vi "Measurement UI.vi"() -> ()   [LabVIEW 2021, in "Crosstalk_Audio ADC_UI.lvlib"]
uses:
  Crosstalk_Audio ADC_UI.lvlib
  Program Files/National Instruments/LabVIEW 2021/examples/Digital Audio Acquisition and Generation Toolkit/subVIs/PCM Interface Type.ctl
  <vilib>/PDM Acquisition Toolkit/shared/controls/Digital Edge.ctl
  shared/Audio ADC Shared.lvlib
  <vilib>/PDM Acquisition Toolkit/shared/PDM Shared.lvlib
panel:
  out "MeasTable":string[][](table)
  in  "MeasGraphs":T1(tab)=enum."Time Domain"
  out "FreqDomainGraph":cluster{"f0":dbl, "df":dbl, dbl[]}(graph) caption="AC"
  out "TimeDomainGraph":waveform(dbl)(graph) caption="AC"
  out "Time domain plot size":i32
  out "Spectrum plot size":i32
  out "dt":dbl
  out "t0":dbl
  out "df":dbl
  out "f0":dbl
  out "Time domain":dbl[](array[numeric])
  out "Spectrum":dbl[](array[numeric])
  out "Crosstalk":dbl
  out "Victim channel name":string
  out "Crosstalk waveform":dbl[](array[numeric])
  out "Frequency waveform":dbl[](array[numeric])
  in  "Victim channel resource name":string
  in  "Digital capture resource name":string
  in  "Configuration tab":enum32{"Protocol", "Measurement"}(tab)
  in  "Frame sync edge for Channel 0":enum16{"Rising", "Falling"}(ring)=enum."Falling"
  in  "Channel count per frame":u8=2
  in  "Channel length":u16=32
  in  "Bit depth":u8=24
  in  "Channel 0 offset":u16=1
  in  "Endianness":enum16{"MSB First", "LSB First"}(ring)
  in  "Data Justification":enum16{"Left Justified", "Right Justified"}(ring) caption="Data justification"
  in  "Frame length":u16=64
  in  "Frame sync pulse width":u16=32
  in  "Bit clock edge sync":enum8{"Rising", "Falling"}(ring)=enum."Falling"
  in  "I2S":bool
  in  "LJ":bool
  in  "RJ":bool
  in  "TDM":bool
  in  "Measurement Duration":dbl=0.1 format="%#_6ps"
  in  "Analog source resource name":string(combo) caption="Resource Name"
  in  "Protocol capture resource name":string(combo) caption="Resource Name"
  in  "Channel Name":string
  in  "Full scale range":dbl=2.825 caption="FULL SCALE RANGE" format="%.3pV"
  in  "Weighting Filter":string(combo)="Linear"
  in  "Data line":u16 caption="Data Line"
  in  "Sample rate":dbl=44100.0 caption="Sample Rate" format="%#.6pHz"
  in  "Measurement settings":string="Measurement Settings"
  in  "Victim amplitude":dbl=1.0 caption="Amplitude" format="%#_6pdB"
  in  "Frequency":dbl=1000.0 format="%#_6pHz"
  in  "Victim channel":dbl=1.0 caption="Vicitim Channel" format="%#_6p"
  in  "Interferer channel":dbl caption="Interferer Channel" format="%#_6p"
  in  "Analog source":string="Analog source"
  in  "Digital capture":string="Digital capture"
  # "Protocols"
  # "PCM data configuration"
  # "Frame sync clock control"
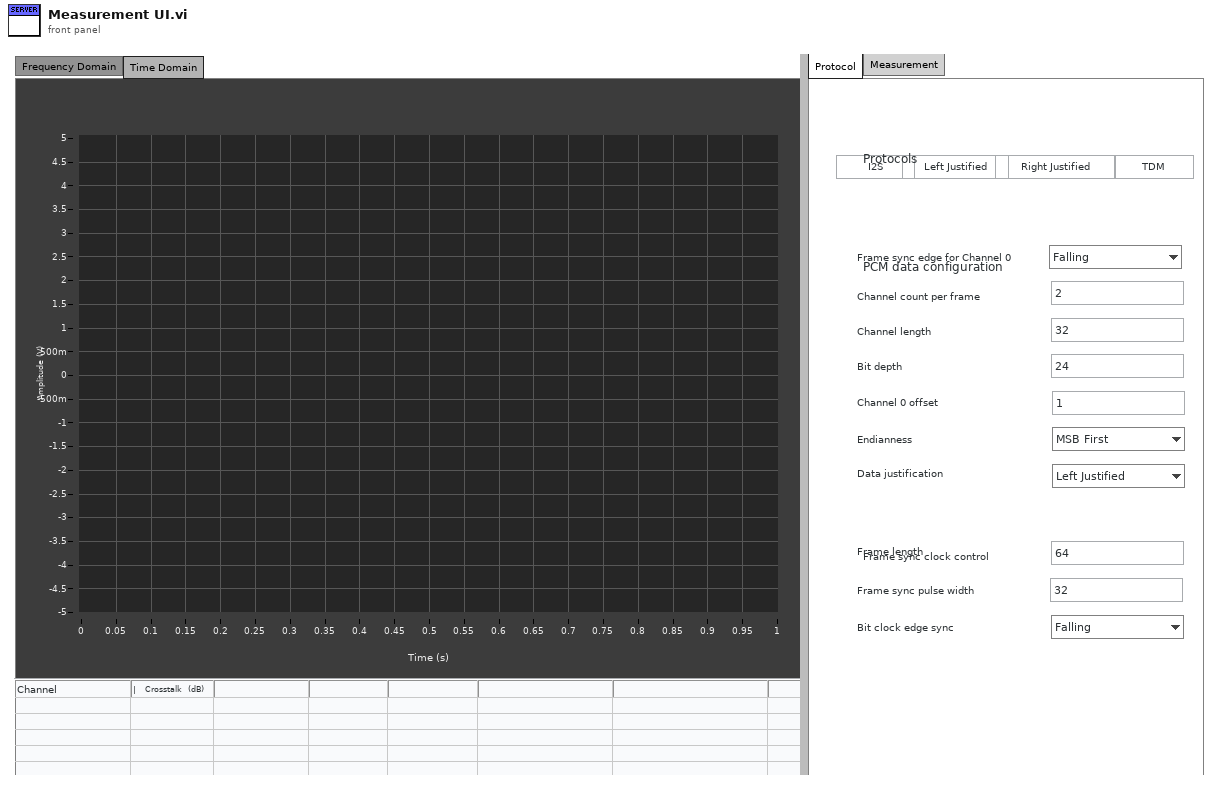
[diagram p1: front panel]
types:
  T1 = enum32{"Frequency Domain", "Time Domain", "Hidden Controls"}
  T2 = typedef "PDM Shared.lvlib/Digital Edge.ctl" = enum8{"Rising", "Falling"}
  T3 = typedef "PCM Interface Type.ctl" = enum16{"I2S", "Left Justified", "Right Justified", "TDM 4 Channel", "TDM 6 Channel", "TDM 8 Channel", "DSP mode", "DSP mode with 1 bit delay", "PCM Short Frame", "PCM Long Frame"}
  T4 = typedef "PDM Shared.lvlib/PCM Frame Sync Control.ctl" = cluster{"Frame Length":u16, "Frame Sync Pulse Width":u16, "Bit Clock Edge  Sync":T2}
  T5 = typedef "PDM Shared.lvlib/PCM Data Format Configuration.ctl" = cluster{"Frame Sync Edge for Channel 0":T2, "Channel Count Per Frame":u8, "Channel Length":u16, "Bit Depth":u8, "Channel 0 Offset":u16, "Endianness":T6, "Data Justification":T7}
  T6 = typedef "PDM Shared.lvlib/PCM Bit Endianness.ctl" = enum16{"MSB First", "LSB First"}
  T7 = typedef "PDM Shared.lvlib/PCM Data Justification.ctl" = enum16{"Left Justified", "Right Justified"}
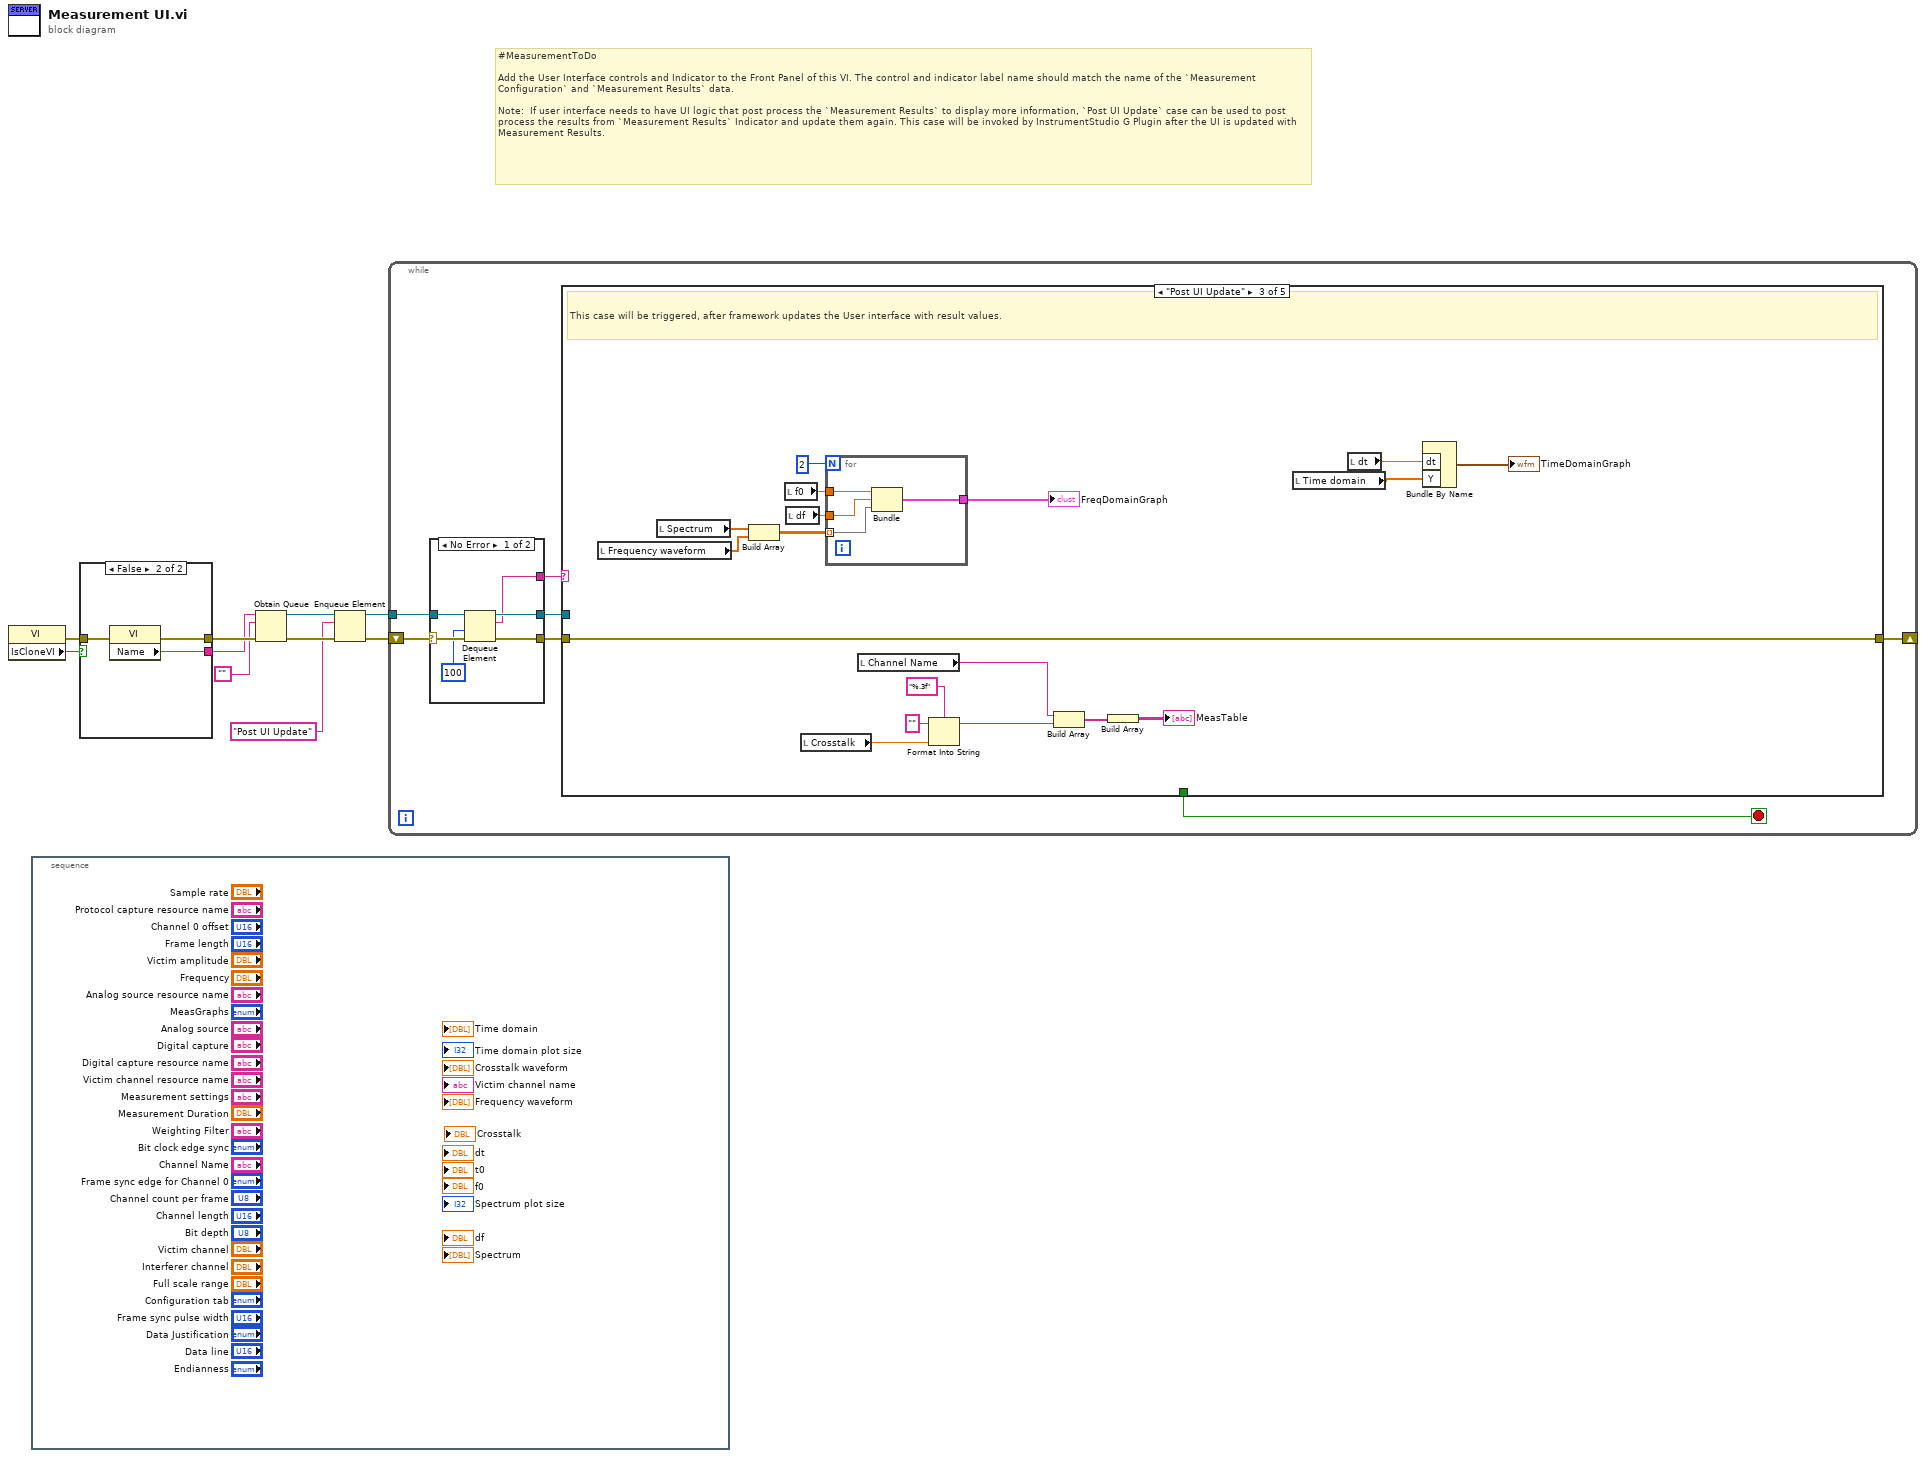
[diagram p0: block diagram]
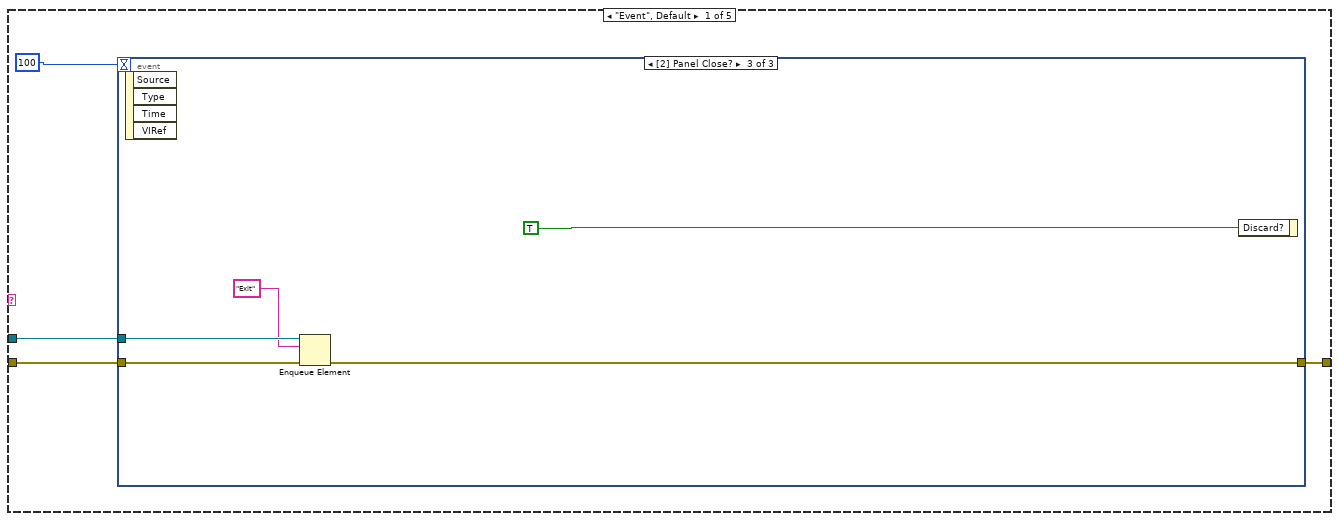
[diagram p2: hidden frame]
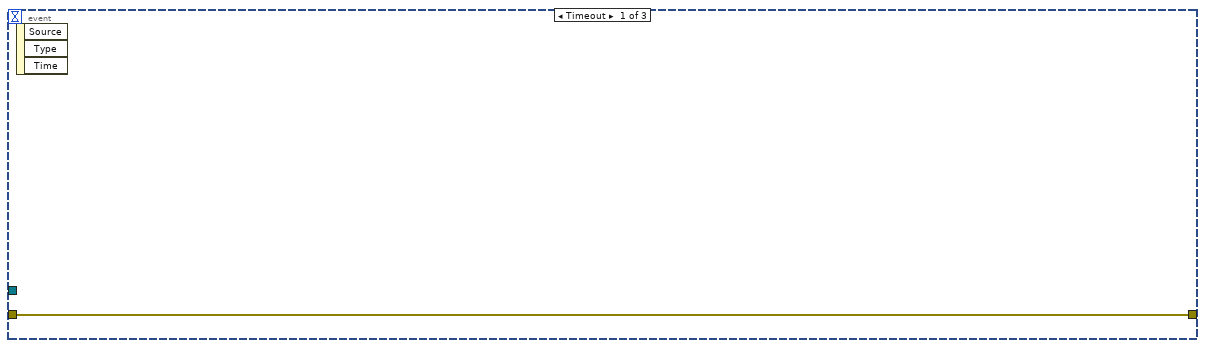
[diagram p3: hidden frame]
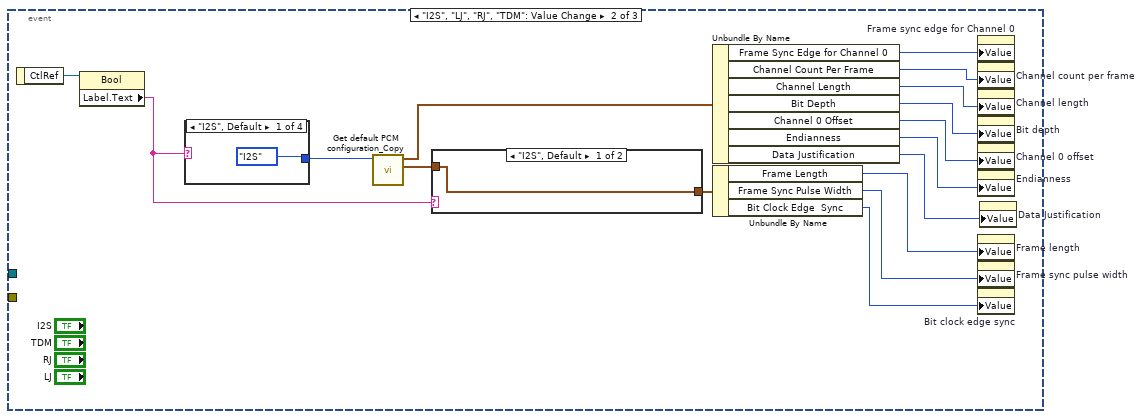
[diagram p4: hidden frame]
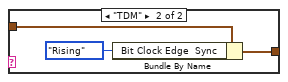
[diagram p5: hidden frame]
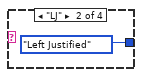
[diagram p6: hidden frame]
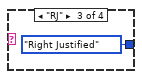
[diagram p7: hidden frame]
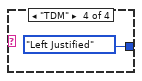
[diagram p8: hidden frame]
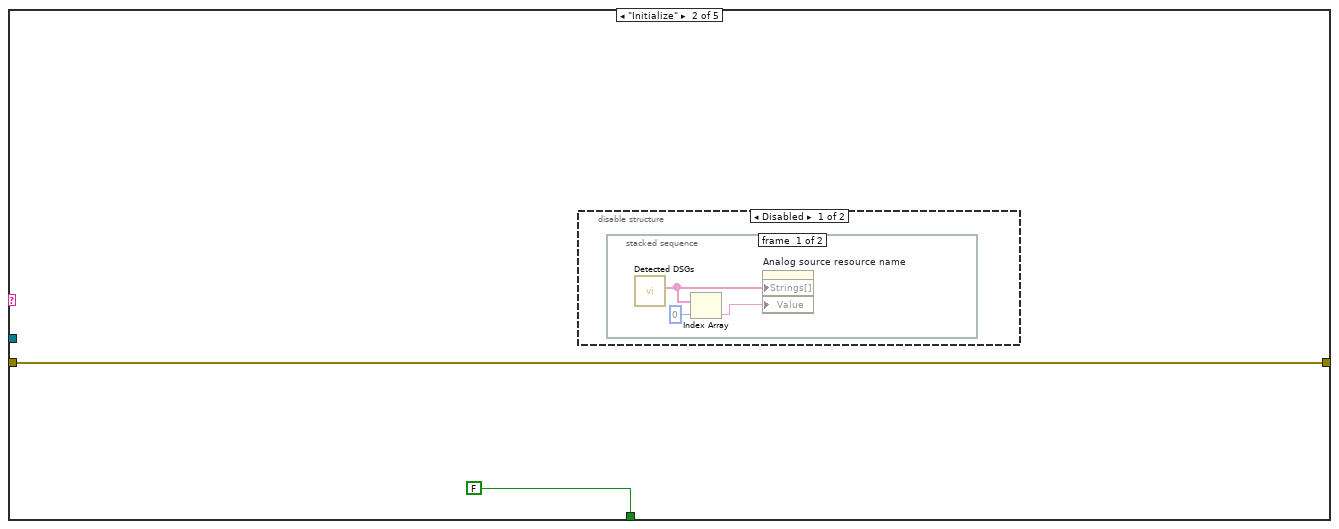
[diagram p9: hidden frame]
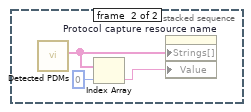
[diagram p10: hidden frame]
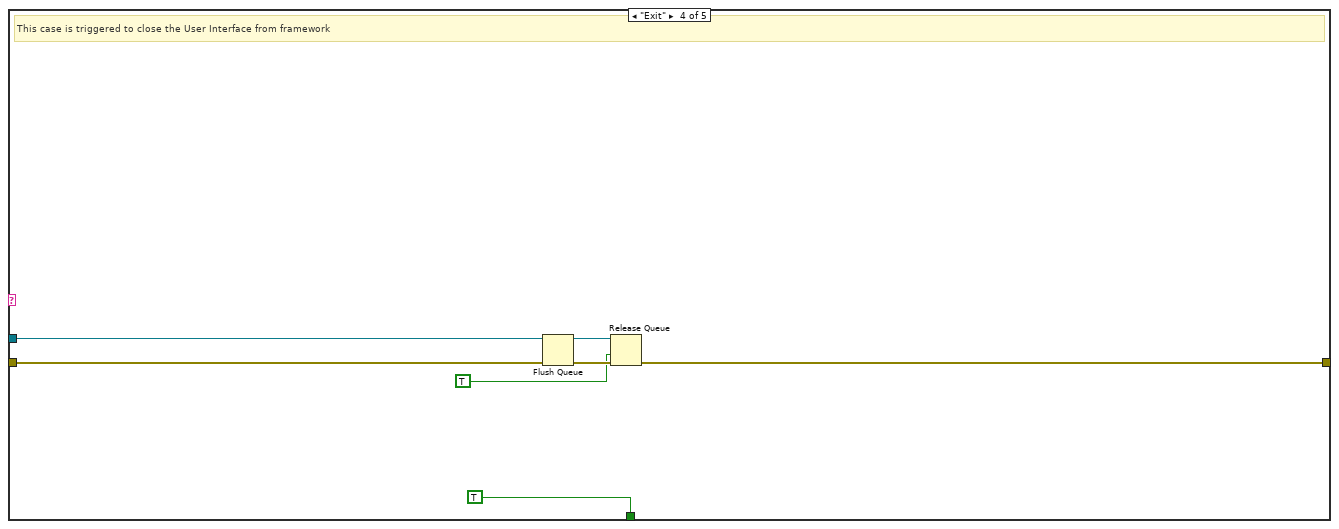
[diagram p12: hidden frame]
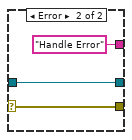
[diagram p14: hidden frame]
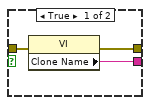
[diagram p15: hidden frame]
diagram:
  # "#MeasurementToDo  \n\nAdd the User Interface controls and Indicator to the Front Panel of this VI. The control and indicator label name should match the name of the `Measurement Configuration` and `Measurement Results` data.\n\nNote:  If user interface needs to have UI logic that post process the `Measurement Results` to display more information, `Post UI Update` case can be used to post process the results from `Measurement Results` Indicator and update them again. This case will be invoked by InstrumentStudio G Plugin after the UI is updated with Measurement Results."
  n1 = property class="VI"() -> (error out=w1:errorcluster, "IsCloneVI"=w2:bool)  [unwired: 2 in, 1 out]
  n2 = stacked-sequence {
    frame #0 {
    }
  }
  n3 = case shown="False" w2 {
    tunnel: [w13 w16] -> w10
    tunnel: [w12 w15] -> w9
    tunnel: w1 -> [w11 w14]
    frame True {
      n4 = property class="VI"(error in=w11) -> (error out=w13:errorcluster, "Clone Name"=w12:string)  [unwired: 1 in, 1 out]
    }
    frame False {
      n5 = property class="VI"(error in=w14) -> (error out=w16:errorcluster, "Name"=w15:string)  [unwired: 1 in, 1 out]
    }
  }
  n6 = Obtain Queue(name (unnamed)=w9, element data type="", error in (no error)=w10) -> (queue out=w6:refnum<queue>, error out=w8:errorcluster)  [unwired: 2 in, 1 out]
  n7 = Enqueue Element(queue=w6, element="Post UI Update", error in (no error)=w8) -> (queue out=w5:refnum<queue>, error out=w7:errorcluster)  [unwired: 1 in, 1 out]
  n8 = while {
    shift-right: [w18] -> _
    shift-left: w7 -> [w23]
    tunnel: w5 -> [w21]
    stop <- w17 stop-if-true
    n9 = case shown="No Error" w23 {
      selector: w23 -> [w101 w104]
      tunnel: [w100 w104] -> w22
      tunnel: w21 -> [w99 w103]
      tunnel: [w98 w103] -> w20
      tunnel: [w97 "Handle Error"] -> w19
      frame No Error {
        n10 = Dequeue Element(queue=w99, timeout in ms (-1)=100, error in (no error)=w101) -> (queue out=w98:refnum<queue>, element=w97:string, error out=w100:errorcluster)  [unwired: 1 out]
      }
      frame Error {
      }
    }
    n11 = case shown="\"Post UI Update\"" w19 {
      tunnel: w22 -> [w26 w59 w70 w94 w95]
      tunnel: w20 -> [w24 _ _ w92 _]
      tunnel: [w27 w59 w70 w89 w95] -> w18
      tunnel: [_ FALSE _ TRUE _] -> w17
      frame "Event", Default {
        n12 = event shown="[2] Panel Close?" {
          selector: _ -> [_ _ _]
          dyn-events: _ -> [_ _ _]
          timeout: 100 -> [_ _ _]
          tunnel: [w28 _ w55] -> w27
          tunnel: w26 -> [w28 _ w56]
          tunnel: w24 -> [_ _ w54]
          event Timeout {
            n13 = event-data() -> ()  [unwired: 1 in, 3 out]
          }
          event "I2S", "LJ", "RJ", "TDM": Value Change {
            n14 = event-data() -> ("CtlRef"=w44:refnum<vi>)  [unwired: 1 in]
            n15 = property class="Bool"(reference=w44) -> ("Label.Text"=w43:string)  [unwired: 1 in, 2 out]
            n16 = case shown="\"I2S\", Default" w43 {
              tunnel: [PCM_Interface_Type."I2S" ("PCM Interfaces") PCM_Interface_Type."Left Justified" ("PCM Interfaces") PCM_Interface_Type."Right Justified" ("PCM Interfaces") PCM_Interface_Type."Left Justified" ("PCM Interfaces")] -> w31
              frame "I2S", Default {
              }
              frame "LJ" {
              }
              frame "RJ" {
              }
              frame "TDM" {
              }
            }
            n17 = call "Get default PCM configuration_Copy.vi"("PCM Interfaces"=w31) -> ("Frame Sync Clock Control"=w29:T4, "PCM Data Configuration"=w30:T5)  [unwired: 9 in]
            n18 = case shown="\"I2S\", Default" w43 {
              tunnel: [w45 w47] -> w42
              tunnel: w29 -> [w45 w46]
              frame "I2S", Default {
              }
              frame "TDM" {
                n19 = Bundle By Name(cluster=w46, "Bit Clock Edge  Sync"=Digital_Edge."Rising") -> (w47:T4)
              }
            }
            n20 = Unbundle By Name(w30) -> ("Frame Sync Edge for Channel 0"=w41:T2, "Channel Count Per Frame"=w40:u8, "Channel Length"=w39:u16, "Bit Depth"=w38:u8, "Channel 0 Offset"=w37:u16, "Endianness"=w36:T6, "Data Justification"=w32:T7)
            n21 = Unbundle By Name(w42) -> ("Frame Length"=w35:u16, "Frame Sync Pulse Width"=w34:u16, "Bit Clock Edge  Sync"=w33:T2)
            n22 = property on="Frame sync edge for Channel 0" class="Enum (strict)"("Value"=w41) -> ()  [unwired: 2 in, 2 out]
            n23 = property on="Channel count per frame" class="DigNum (strict)"("Value"=w40) -> ()  [unwired: 2 in, 2 out]
            n24 = property on="Channel length" class="DigNum (strict)"("Value"=w39) -> ()  [unwired: 2 in, 2 out]
            n25 = property on="Bit depth" class="DigNum (strict)"("Value"=w38) -> ()  [unwired: 2 in, 2 out]
            n26 = property on="Channel 0 offset" class="DigNum (strict)"("Value"=w37) -> ()  [unwired: 2 in, 2 out]
            n27 = property on="Endianness" class="Enum (strict)"("Value"=w36) -> ()  [unwired: 2 in, 2 out]
            n28 = property on="Frame length" class="DigNum (strict)"("Value"=w35) -> ()  [unwired: 2 in, 2 out]
            n29 = property on="Frame sync pulse width" class="DigNum (strict)"("Value"=w34) -> ()  [unwired: 2 in, 2 out]
            n30 = property on="Bit clock edge sync" class="Enum (strict)"("Value"=w33) -> ()  [unwired: 2 in, 2 out]
            n31 = property on="Data Justification" class="Enum (strict)"("Value"=w32) -> ()  [unwired: 2 in, 2 out]
          }
          event Panel Close? {
            n32 = event-data() -> ()  [unwired: 1 in, 4 out]
            n33 = Enqueue Element(queue=w54, element="Exit", error in (no error)=w56) -> (error out=w55:errorcluster)  [unwired: 1 in, 2 out]
            n34 = event-data("Discard?"=TRUE) -> ()  [unwired: 1 in, 1 out]
          }
        }
      }
      frame "Initialize" {
        n35 = disable-structure shown="Disabled" {
          frame Disabled {
            n36 = stacked-sequence {
              frame #0 {
                n37 = call "Detected DSGs.vi"() -> ("AO channels"=w62:string[])  [unwired: 11 in]
                n38 = Index Array(array=w62, index=0) -> (element=w61:string)
                n39 = property on="Analog source resource name" class="CmbBox"("Strings[]"=w62, "Value"=w61) -> ()  [unwired: 2 in, 2 out]
              }
              frame #1 {
                n40 = call "Detected PDMs.vi"() -> ("PDM devices"=w65:string[])  [unwired: 11 in]
                n41 = Index Array(array=w65, index=0) -> (element=w64:string)
                n42 = property on="Protocol capture resource name" class="CmbBox"("Strings[]"=w65, "Value"=w64) -> ()  [unwired: 2 in, 2 out]
              }
            }
          }
          frame Enabled {
          }
        }
      }
      frame "Post UI Update" {
        # "This case will be triggered, after framework updates the User interface with result values."
        n43 = local read "Frequency waveform"() -> (w79:dbl[])
        n44 = local read "Spectrum"() -> (w81:dbl[])
        n45 = Build Array(w81, w79) -> (w69:dbl[][])
        n46 = local read "f0"() -> (w82:dbl)
        n47 = local read "df"() -> (w80:dbl)
        n48 = local read "Crosstalk"() -> (w66:dbl)
        n49 = for {
          N: 2 -> [_]
          tunnel: w82 -> [w87]
          tunnel: w80 -> [w86]
          tunnel: [w85] -> w68
          tunnel: w69 -> [w84] mode=indexing
          n50 = Bundle("f0"=w87, "df"=w86, w84) -> (w85:cluster{"f0":dbl, "df":dbl, dbl[]})  [unwired: 1 in]
        }
        "FreqDomainGraph" <- w68
        n51 = local read "Channel Name"() -> (w73:string)
        n52 = Format Into String(format string="%.3f", initial string="", w66) -> (resulting string=w74:string)  [unwired: 1 in, 1 out]
        n53 = Build Array(w73, w74) -> (w72:string[])
        n54 = Build Array(w72) -> (→"MeasTable":string[][])
        n55 = local read "Time domain"() -> (w77:dbl[])
        n56 = local read "dt"() -> (w78:dbl)
        n57 = Bundle By Name("dt"=w78, "Y"=w77) -> (→"TimeDomainGraph":waveform(dbl))  [unwired: 1 in]
      }
      frame "Exit" {
        # "This case is triggered to close the User Interface from framework"
        n58 = Flush Queue(queue=w92, error in (no error)=w94) -> (queue out=w91:refnum<queue>, error out=w90:errorcluster)  [unwired: 1 out]
        n59 = Release Queue(queue=w91, force destroy? (F)=TRUE, error in (no error)=w90) -> (error out=w89:errorcluster)  [unwired: 2 out]
      }
      frame "Handle Error" {
      }
    }
  }
